vi "Append Inheritance.vi"(9 "Class":string, 10 "Parent Class":refnum<vi>, 11 "Class Relations Map":T1(c390)) -> (3 "Class Relations Map Out":T1(c390))   [LabVIEW 2019]
uses:
  <vilib>/Utility/miscctls.llb/LVMapReplaceAction.ctl
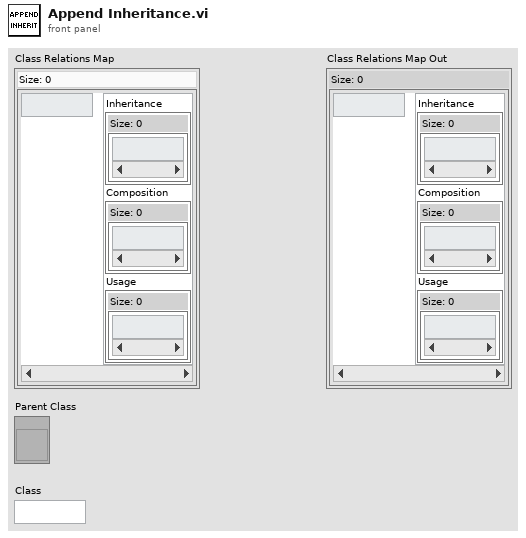
[diagram p1: front panel]
types:
  T1 = map{string, cluster{"Inheritance":set{string}, "Composition":set{string}, "Usage":set{string}}}
  T2 = typedef "LVMapReplaceAction.ctl" = enum32{"Modify Entry only if found", "Add or Modify Entry", "Delete Entry"}
  T3 = cluster{"Inheritance":set{string}, "Composition":set{string}, "Usage":set{string}}
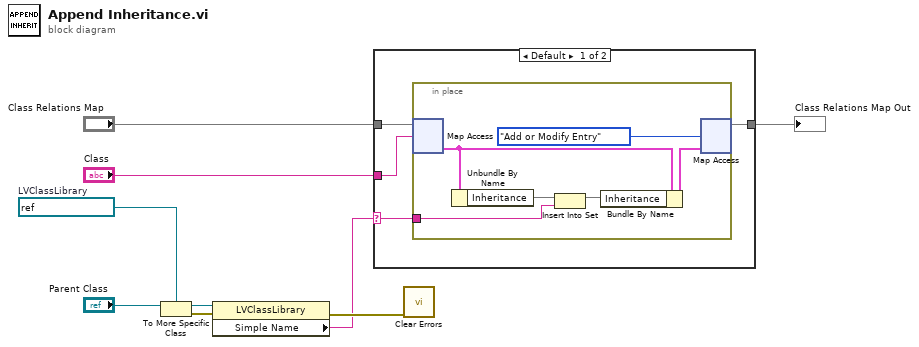
[diagram p0: block diagram]
diagram:
  w7 = refnum<vi> refnum  # LVClassLibrary
  n1 = To More Specific Class(target class=w7, reference="Parent Class") -> (specific class reference=w2:refnum<vi>, error out=w4:errorcluster)  [unwired: 1 in]
  n2 = property class="LVClassLibrary"(reference=w2, error in=w4) -> (error out=w3:errorcluster, "Simple Name"=w1:string)  [unwired: 1 out]
  n3 = case shown="Default" w1 {
    selector: w1 -> [w10 _]
    tunnel: [w12 w20] -> w5
    tunnel: "Class Relations Map" -> [w13 w20]
    tunnel: "Class" -> [w11 _]
    frame Default {
      n4 = in-place {
        in-place-border: w10 -> [w14]
        n5 = in-place-map #1(w13, w11) -> (w18:T3)  [unwired: 1 in, 1 out]
        n6 = Unbundle By Name(w18) -> ("Inheritance"=w16:set{string})
        n7 = Insert Into Set(10:w14, 11:w16) -> (3:w15:set{string})  [unwired: 1 out]
        n8 = Bundle By Name(cluster=w18, "Inheritance"=w15) -> (w17:T3)
        n9 = in-place-map #1(w17, LVMapReplaceAction."Add or Modify Entry" ("action")) -> (w12:T1)  [unwired: 2 out]
      }
    }
    frame "" {
    }
  }
  "Class Relations Map Out" <- w5
  n10 = call <vilib>:"Clear Errors.vi"("error in (no error)"=w3) -> ()  [unwired: 5 in, 2 out]
